vi "卫星模拟器自动控制软件.vi"() -> ()   [LabVIEW 2012]
uses:
  <vilib>/Utility/error.llb/DialogType.ctl
  <vilib>/DAQmx/create/channels.llb/DAQmx Create Channel (DO-Digital Output).vi
  <vilib>/vision/NI_Vision_Development_Module.lvlib
panel:
  in  "缩放比例 (像素/cm)":dbl=4.099468
  in  "远程数据记录器传输状态":bool
  in  "是否下传定位点信息":bool
  in  "远程端口":u16=61557
  in  "本地端口":u16=61556
  in  "远程终端地址":string="localhost"
  in  "broadcast":bool
  in  "是否姿态保持":bool
  out "alpha":dbl
  out "定位点信息":T1(array[cluster]) {"Aspect Ratio" format="%.2f"; "Orientation" format="%.2f"; "Area" format="%.2f"; "Object Center"."Y" format="%.2f"; "Object Center"."X" format="%.2f"}
  in  "Y中心校正":dbl
  in  "X中心校正":dbl
  out "相对偏角(deg)":dbl
  in  "目标Y":dbl
  in  "目标X":dbl
  out "X速率(cm/s)":dbl
  out "Y速率(cm/s)":dbl
  in  "OK Button":bool
  out "角速度(deg/s)":dbl
  in  "气浮状态":bool
  in  "控制频率(Hz)":u32=20
  in  "目标偏角":dbl
  in  "STOP":bool caption="stop (F)"
  out "导航相机输出":T2(plugin-control)
  out "alpha (deg)":dbl
  out "X偏移量 (cm)":dbl
  out "Y偏移量 (cm)":dbl
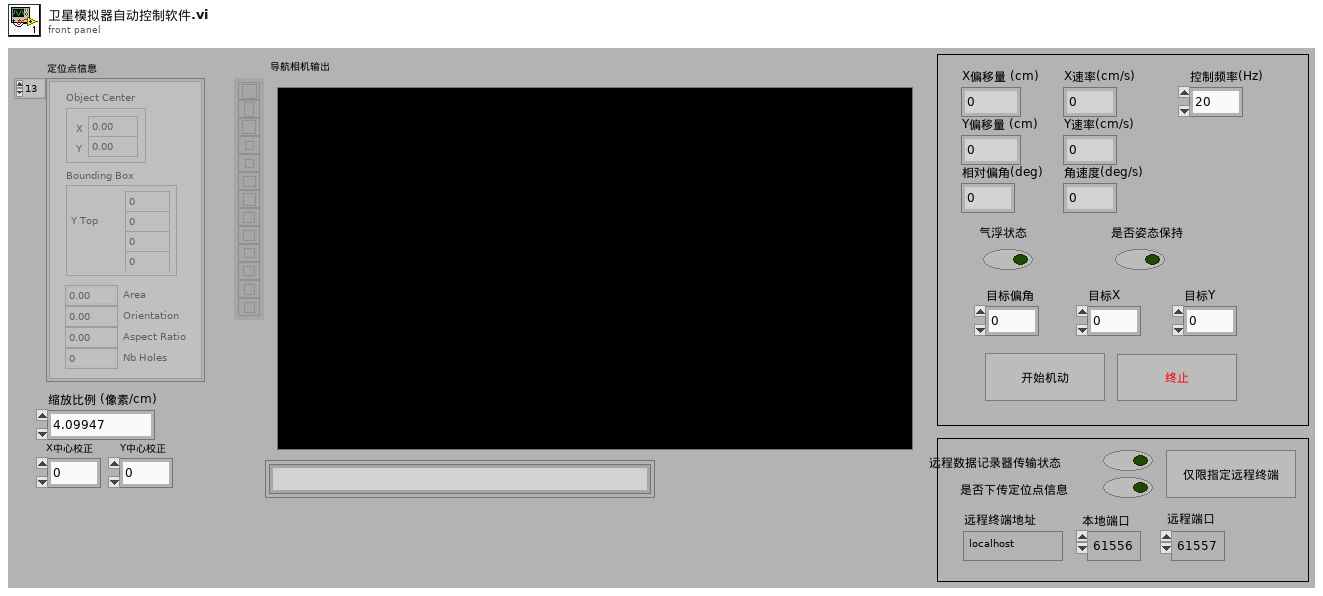
[diagram p1: front panel]
types:
  T1 = cluster{"Object Center":cluster{"X":sgl, "Y":sgl}, "Bounding Box":cluster{"X Left":i32, "Y Top":i32, "X Right":i32, "Y Bottom":i32}, "Area":sgl, "Orientation":sgl, "Aspect Ratio":sgl, "Nb Holes":i32}[]
  T2 = typedef "IMAQ Image.ctl" = refnum<image>
  T3 = typedef "DialogType.ctl" = u16
  T4 = cluster{"X偏移量 (cm)":dbl, "Y偏移量 (cm)":dbl, "相对偏角(deg)":dbl}
  T5 = cluster{"Objects":u16, "Threshold":i32, "Reject Border":bool, "Fill Holes":bool, "Min Object Size":bool, "Min Size":i32, "Max Object Size":bool, "Max Size":i32, "Show Search Area":bool, "Show Center":bool, "Show Bounding Box":bool}
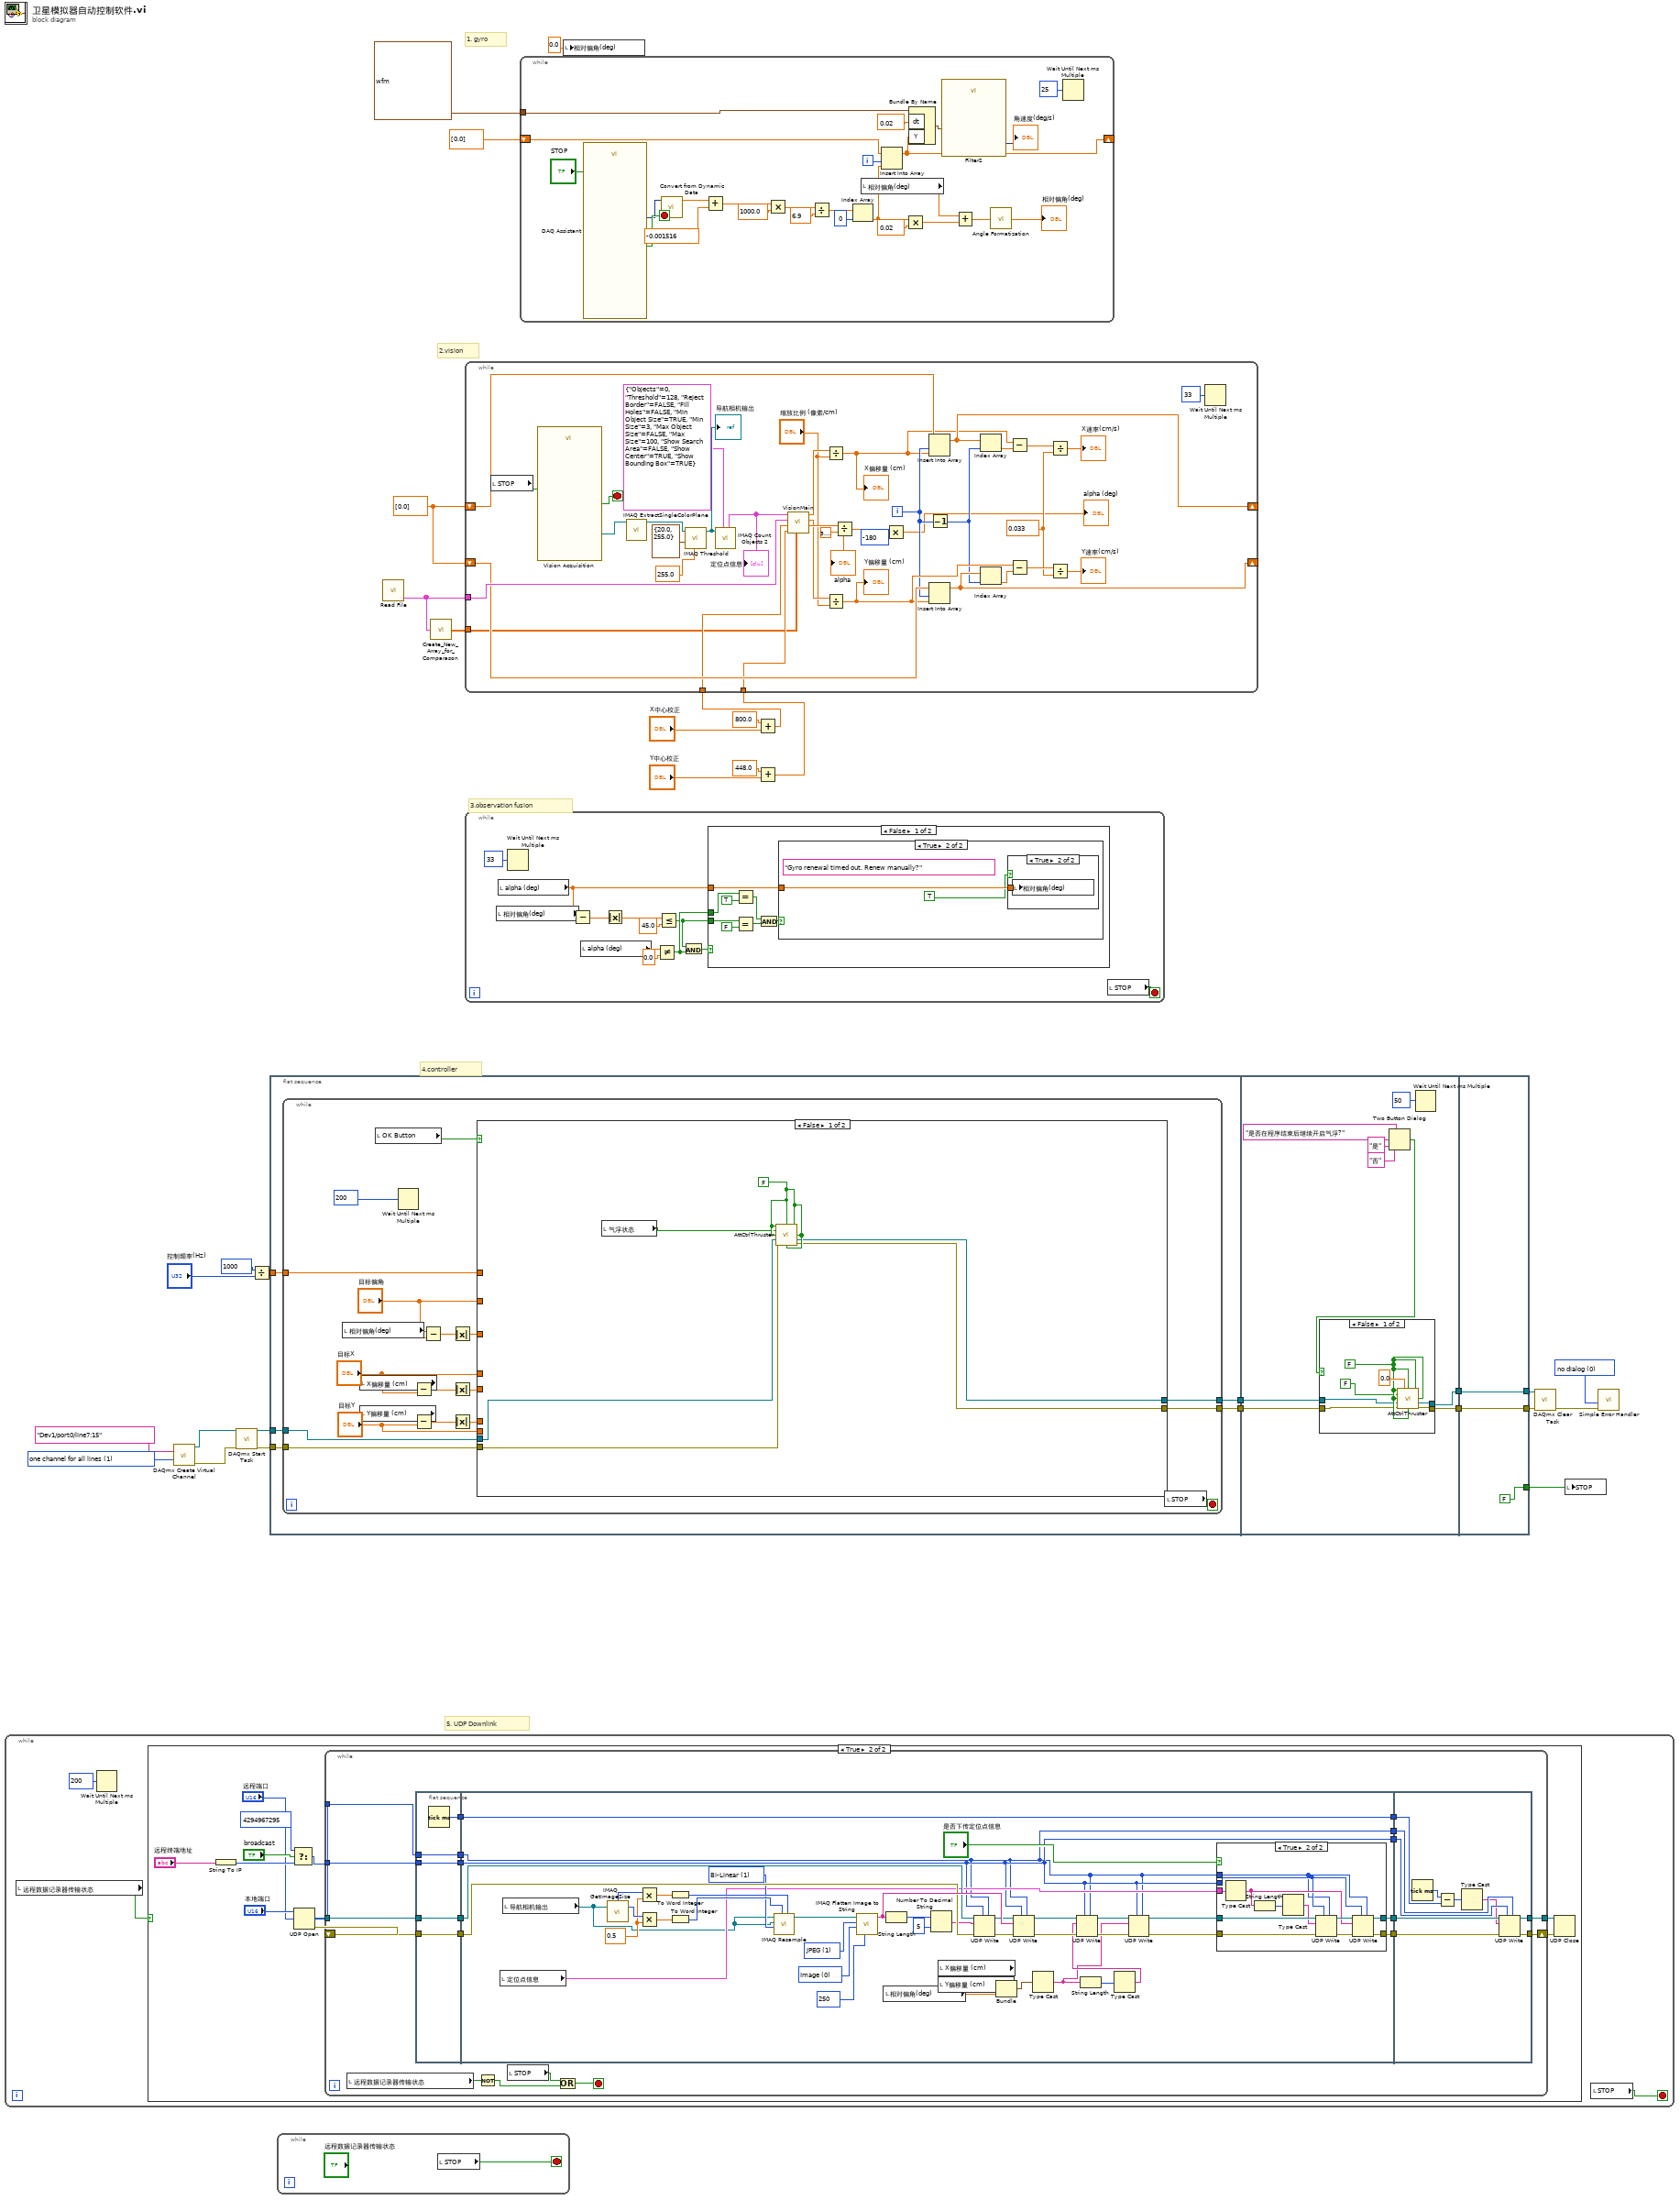
[diagram p0: block diagram]
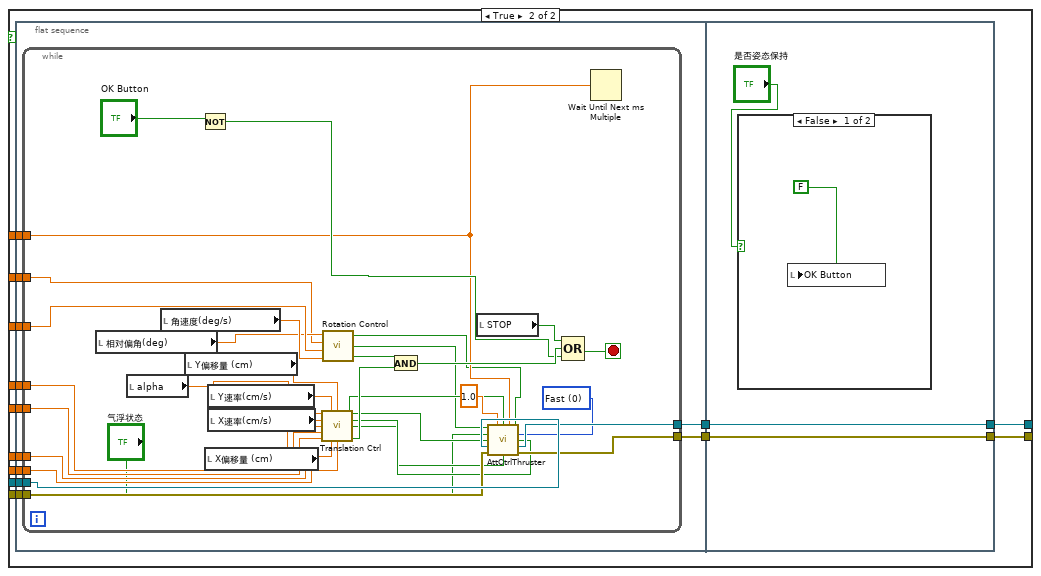
[diagram p4: hidden frame]
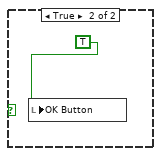
[diagram p5: hidden frame]
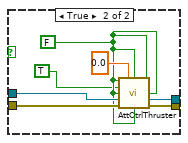
[diagram p6: hidden frame]
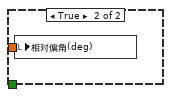
[diagram p9: hidden frame]
diagram:
  w25 = T3 0 items=["no dialog", "OK message", "continue or stop message", "OK message + warnings", "continue/stop + warnings"] ("type of dialog (OK msg:1)")
  w28 = 1 items=["one channel for each line", "one channel for all lines"] ("line grouping")
  w12 = dbl[] [0.0]
  # "5. UDP Downlink"
  # "4.controller"
  # "3.observation fusion"
  # "2.vision"
  # "1. gyro"
  n1 = while {
    stop <- w32 stop-if-true
    n2 = local read "远程数据记录器传输状态"() -> (w33:bool)
    n3 = Wait Until Next ms Multiple(millisecond multiple=u32 200) -> ()  [unwired: 1 out]
    n4 = case shown="True" w33 {
      frame False {
      }
      frame True {
        n5 = String To IP(1:"远程终端地址") -> (0:w41:u32)
        n6 = Select(t=u32 4294967295, s="broadcast", f=w41) -> (s? t:f=w38:u32)
        n7 = UDP Open(11:"本地端口") -> (port=w37:refnum<k16>, 0:w36:errorcluster)  [unwired: 1 in, 4 out]
        n8 = while {
          tunnel: "远程端口" -> [w64]
          tunnel: w38 -> [w63]
          tunnel: w37 -> [w62]
          tunnel: [w60] -> w35
          shift-right: [w59] -> w34
          shift-left: w36 -> [w61]
          stop <- w48 stop-if-true
          n9 = local read "远程数据记录器传输状态"() -> (w46:bool)
          n10 = flat-sequence {
            tunnel: w62 -> [w66]
            tunnel: w64 -> [w67]
            tunnel: w63 -> [w68]
            tunnel: w61 -> [w69]
            tunnel: [w69] -> w58
            tunnel: [w68] -> w57
            tunnel: [w67] -> w56
            tunnel: [w66] -> w55
            tunnel: [w65] -> w54
            tunnel: [w89] -> w53
            tunnel: [w88] -> w52
            tunnel: w58 -> [w107]
            tunnel: w57 -> [w71]
            tunnel: w56 -> [w70]
            tunnel: w55 -> [w91]
            tunnel: [w90] -> w51
            tunnel: w54 -> [w90]
            tunnel: [w70] -> w50
            tunnel: [w71] -> w49
            tunnel: [w131] -> w60
            tunnel: [w125] -> w59
            tunnel: w53 -> [w126]
            tunnel: w52 -> [w132]
            tunnel: w51 -> [w133]
            tunnel: w50 -> [w130]
            tunnel: w49 -> [w129]
            frame #0 {
              n11 = Tick Count (ms)() -> (millisecond timer value=w65:u32)
            }
            frame #1 {
              w95 = u32 1 items=["Zero Order", "Bi-Linear", "Quadratic", "Cubic Spline"] ("Interpolation Type")
              w96 = 0.5
              w104 = 0 items=["Image", "Image and Vision Info", "Reference to Image"] ("Type of Flatten (Image and Vision Info)")
              w109 = 1 items=["None", "JPEG", "PACKED BINARY"] ("Compression (None)")
              n12 = local read "定位点信息"() -> (w86:T1)
              n13 = local read "导航相机输出"() -> (w85:T2)
              n14 = call "IMAQ GetImageSize"("Image"=w85) -> ("Y Resolution"=w97:i32, "X Resolution"=w98:i32)  [unwired: 3 in, 1 out]
              n15 = Multiply(x=w98, y=w96) -> (x*y=w100:dbl)
              n16 = Multiply(x=w97, y=w96) -> (x*y=w102:dbl)
              n17 = To Word Integer(number=w100) -> (16bit integer=w99:i16)
              n18 = To Word Integer(number=w102) -> (16bit integer=w101:i16)
              n19 = call "IMAQ Resample"("X Resolution"=w99, "Y Resolution"=w101, "Interpolation Type"=w95, "Image Dst"=w85, "Image Src"=w85) -> ("Image Dst Out"=w103:T2)  [unwired: 5 in, 1 out]
              n20 = call "IMAQ Flatten Image to String"("Quality (750)"=250, "Type of Flatten (Image and Vision Info)"=w104, "Compression (None)"=w109, "Image"=w103) -> ("Data String"=w108:string)  [unwired: 6 in, 1 out]
              n21 = local read "相对偏角(deg)"() -> (w82:dbl)
              n22 = String Length(string=w108) -> (length=w94:i32)
              n23 = Number To Decimal String(number=w94, width (-)=i16 5) -> (decimal integer string=w93:string)
              n24 = local read "X偏移量 (cm)"() -> (w84:dbl)
              n25 = local read "Y偏移量 (cm)"() -> (w83:dbl)
              n26 = UDP Write(address=w71, port or service name=w70, connection ID=w91, data in=w93, 8:w107) -> (error out=w106:errorcluster, 3:w105:refnum<k16>)  [unwired: 1 out]
              n27 = Bundle("X偏移量 (cm)"=w84, "Y偏移量 (cm)"=w83, "相对偏角(deg)"=w82) -> (w81:T4)  [unwired: 1 in]
              n28 = UDP Write(address=w71, port or service name=w70, connection ID=w105, data in=w108, 8:w106) -> (error out=w79:errorcluster, 3:w80:refnum<k16>)  [unwired: 1 out]
              n29 = Type Cast(x=w81) -> (*(type *) &x=w72:string)  [unwired: 1 in]
              n30 = String Length(string=w72) -> (length=w74:i32)
              n31 = Type Cast(x=w74) -> (*(type *) &x=w73:string)  [unwired: 1 in]
              n32 = UDP Write(address=w71, port or service name=w70, connection ID=w80, data in=w73, 8:w79) -> (error out=w78:errorcluster, 3:w76:refnum<k16>)  [unwired: 1 out]
              n33 = UDP Write(address=w71, port or service name=w70, connection ID=w76, data in=w72, 8:w78) -> (error out=w77:errorcluster, 3:w75:refnum<k16>)  [unwired: 1 out]
              n34 = case shown="True" "是否下传定位点信息" {
                tunnel: w86 -> [_ w124]
                tunnel: w77 -> [w112 w122]
                tunnel: [w112 w120] -> w89
                tunnel: w75 -> [w111 w119]
                tunnel: [w111 w117] -> w88
                tunnel: w71 -> [_ w114]
                tunnel: w70 -> [_ w113]
                frame False {
                }
                frame True {
                  n35 = Type Cast(x=w124) -> (*(type *) &x=w115:string)  [unwired: 1 in]
                  n36 = String Length(string=w115) -> (length=w123:i32)
                  n37 = Type Cast(x=w123) -> (*(type *) &x=w116:string)  [unwired: 1 in]
                  n38 = UDP Write(address=w114, port or service name=w113, connection ID=w119, data in=w116, 8:w122) -> (error out=w121:errorcluster, 3:w118:refnum<k16>)  [unwired: 1 out]
                  n39 = UDP Write(address=w114, port or service name=w113, connection ID=w118, data in=w115, 8:w121) -> (error out=w120:errorcluster, 3:w117:refnum<k16>)  [unwired: 1 out]
                }
              }
            }
            frame #2 {
              n40 = Tick Count (ms)() -> (millisecond timer value=w134:u32)
              n41 = Subtract(x=w134, y=w133) -> (x-y=w128:u32)
              n42 = Type Cast(x=w128) -> (*(type *) &x=w127:string)  [unwired: 1 in]
              n43 = UDP Write(address=w129, port or service name=w130, connection ID=w132, data in=w127, 8:w126) -> (error out=w125:errorcluster, 3:w131:refnum<k16>)  [unwired: 1 out]
            }
          }
          n44 = Not(x=w46) -> (.not. x?=w45:bool)
          n45 = local read "STOP"() -> (w47:bool)
          n46 = Or(x=w47, y=w45) -> (x .or. y?=w48:bool)
        }
        n47 = UDP Close(connection ID=w35, 8:w34) -> ()  [unwired: 2 out]
      }
    }
    n48 = local read "STOP"() -> (w32:bool)
  }
  n49 = call-poly <vilib>:"DAQmx Create Virtual Channel.vi"("lines"=tag "Dev1/port0/line7:15" ("Lines"), "line grouping"=w28) -> ("task out"=w26:refnum<k21>, "error out"=w27:errorcluster)  [unwired: 12 in]
  n50 = call <vilib>:"DAQmx Start Task.vi"("task/channels in"=w26, "error in"=w27) -> ("task out"=w21:refnum<k21>, "error out"=w20:errorcluster)  [unwired: 12 in]
  n51 = Divide(x=u32 1000 ("milliseconds to wait"), y="控制频率(Hz)") -> (x/y=w17:dbl)
  n52 = flat-sequence {
    tunnel: w21 -> [w139]
    tunnel: w20 -> [w138]
    tunnel: w17 -> [w135]
    tunnel: [w137] -> w16
    tunnel: [w136] -> w15
    tunnel: w16 -> [w237]
    tunnel: w15 -> [w235]
    tunnel: [w236] -> w5
    tunnel: [w234] -> w4
    tunnel: [w253] -> w18
    tunnel: [w254] -> w19
    tunnel: w5 -> [w254]
    tunnel: w4 -> [w253]
    tunnel: [FALSE] -> w3
    frame #0 {
      n53 = while {
        tunnel: w139 -> [w159]
        tunnel: w138 -> [w158]
        tunnel: [w157] -> w137
        tunnel: [w156] -> w136
        tunnel: w135 -> [w141]
        stop <- w155 stop-if-true
        n54 = local read "相对偏角(deg)"() -> (w154:dbl)
        n55 = local read "X偏移量 (cm)"() -> (w150:dbl)
        n56 = local read "Y偏移量 (cm)"() -> (w146:dbl)
        n57 = local read "OK Button"() -> (w142:bool)
        n58 = Wait Until Next ms Multiple(millisecond multiple=200) -> ()  [unwired: 1 out]
        n59 = Subtract(x=w150, y="目标X") -> (x-y=w148:dbl)
        n60 = Subtract(x=w146, y="目标Y") -> (x-y=w144:dbl)
        n61 = Subtract(x=w154, y="目标偏角") -> (x-y=w152:dbl)
        n62 = Absolute Value(x=w152) -> (abs(x)=w151:dbl)
        n63 = Absolute Value(x=w148) -> (abs(x)=w147:dbl)
        n64 = Absolute Value(x=w144) -> (abs(x)=w143:dbl)
        n65 = case shown="False" w142 {
          tunnel: w159 -> [w163 w178]
          tunnel: w158 -> [w162 w177]
          tunnel: [w160 w176] -> w157
          tunnel: [w161 w175] -> w156
          tunnel: w141 -> [_ w174]
          tunnel: "目标偏角" -> [_ w173]
          tunnel: w151 -> [_ w172]
          tunnel: "目标X" -> [_ w171]
          tunnel: w147 -> [_ w170]
          tunnel: "目标Y" -> [_ w169]
          tunnel: w143 -> [_ w168]
          frame False {
            w165 = FALSE
            n66 = local read "气浮状态"() -> (w164:bool)
            n67 = call "AttCtrlThruster.vi"("ctclk"=w165, "Up"=w165, "clkwis"=w165, "Float"=w164, "Left"=w165, "Right"=w165, "task in"=w163, "error in"=w162, "Down"=w165) -> ("task out"=w161:refnum<k21>, "error out"=w160:errorcluster)  [unwired: 5 in]
          }
          frame True {
            n68 = flat-sequence {
              tunnel: w178 -> [w189]
              tunnel: w177 -> [w188]
              tunnel: w174 -> [w185]
              tunnel: w173 -> [w184]
              tunnel: w172 -> [w183]
              tunnel: w171 -> [w182]
              tunnel: w170 -> [w181]
              tunnel: w169 -> [w180]
              tunnel: w168 -> [w179]
              tunnel: [w187] -> w167
              tunnel: [w186] -> w166
              tunnel: [w225] -> w175
              tunnel: [w226] -> w176
              tunnel: w167 -> [w226]
              tunnel: w166 -> [w225]
              frame #0 {
                n69 = while {
                  tunnel: w189 -> [w223]
                  tunnel: w188 -> [w222]
                  tunnel: [w220] -> w187
                  tunnel: [w221] -> w186
                  tunnel: w185 -> [w193]
                  tunnel: w184 -> [w201]
                  tunnel: w183 -> [w216]
                  tunnel: w182 -> [w200]
                  tunnel: w181 -> [w211]
                  tunnel: w180 -> [w199]
                  tunnel: w179 -> [w198]
                  stop <- w217 stop-if-true
                  w207 = u16 0 items=["Fast", "Slow"] ("Angular Acceleration")
                  n70 = local read "相对偏角(deg)"() -> (w214:dbl)
                  n71 = local read "alpha"() -> (w195:dbl)
                  n72 = local read "角速度(deg/s)"() -> (w215:dbl)
                  n73 = local read "Y偏移量 (cm)"() -> (w209:dbl)
                  n74 = Not(x="OK Button") -> (.not. x?=w196:bool)
                  n75 = local read "X偏移量 (cm)"() -> (w212:dbl)
                  n76 = local read "Y速率(cm/s)"() -> (w210:dbl)
                  n77 = local read "X速率(cm/s)"() -> (w213:dbl)
                  n78 = call "Translation Ctrl.vi"("Alpha"=w195, "Filtered Speed Y"=w210, "Y In"=w209, "Filtered Speed X"=w213, "X In"=w212, "X Desired"=w200, "Original Difference X"=w211, "Original Difference Y"=w198, "Y Desired"=w199) -> ("Left"=w205:bool, "Right"=w204:bool, "Down"=w203:bool, "Up"=w202:bool, "Maneuver Complete?"=w206:bool)  [unwired: 2 in]
                  n79 = call "Rotation Control.vi"("Filtered Ohmega"=w215, "Original Difference"=w216, "Alpha Desired"=w201, "Alpha In"=w214) -> ("Maneuver Complete?"=w194:bool, "Counter-ClkWise Rot Ctrl"=w190:bool, "Clockwise Rot Ctrl"=w191:bool)
                  n80 = And(x=w194, y=w206) -> (x .and. y?=w208:bool)
                  n81 = local read "STOP"() -> (w218:bool)
                  n82 = call "AttCtrlThruster.vi"("ctclk"=w190, "Duty Cycle"=1.0, "Up"=w202, "Period"=w193, "clkwis"=w191, "Float"="气浮状态", "Angular Acceleration"=w207, "Left"=w205, "Right"=w204, "task in"=w223, "error in"=w222, "Down"=w203) -> ("task out"=w221:refnum<k21>, "error out"=w220:errorcluster)  [unwired: 2 in]
                  n83 = Compound Arithmetic op=OR(w218, w208, w196) -> (w217:bool)
                  n84 = Wait Until Next ms Multiple(millisecond multiple=w193) -> ()  [unwired: 1 out]
                }
              }
              frame #1 {
                n85 = case shown="False" "是否姿态保持" {
                  frame False {
                    n86 = local write "OK Button"(FALSE) -> ()
                  }
                  frame True {
                    n87 = local write "OK Button"(TRUE) -> ()
                  }
                }
              }
            }
          }
        }
        n88 = local read "STOP"() -> (w155:bool)
      }
    }
    frame #1 {
      n89 = Two Button Dialog(message="是否在程序结束后继续开启气浮?", 1:"否" ("F button name (\"Cancel\")"), 2:"是" ("T button name (\"OK\")")) -> (T button?=w231:bool)
      n90 = case shown="False" w231 {
        tunnel: w237 -> [w240 w251]
        tunnel: [w238 w250] -> w236
        tunnel: w235 -> [w241 w249]
        tunnel: [w239 w248] -> w234
        frame False {
          w243 = FALSE
          n91 = call "AttCtrlThruster.vi"("ctclk"=w243, "Duty Cycle"=0.0, "Up"=w243, "clkwis"=w243, "Float"=FALSE, "Left"=w243, "Right"=w243, "task in"=w241, "error in"=w240, "Down"=w243) -> ("task out"=w239:refnum<k21>, "error out"=w238:errorcluster)  [unwired: 4 in]
        }
        frame True {
          w246 = FALSE
          n92 = call "AttCtrlThruster.vi"("ctclk"=w246, "Duty Cycle"=0.0, "Up"=w246, "clkwis"=w246, "Float"=TRUE, "Left"=w246, "Right"=w246, "task in"=w249, "error in"=w251, "Down"=w246) -> ("task out"=w248:refnum<k21>, "error out"=w250:errorcluster)  [unwired: 4 in]
        }
      }
      n93 = Wait Until Next ms Multiple(millisecond multiple=u32 50) -> ()  [unwired: 1 out]
    }
    frame #2 {
    }
  }
  n94 = while {
    stop <- w255 stop-if-true
    n95 = local read "STOP"() -> (w255:bool)
  }
  n96 = call "Read File.vi"() -> ("Objects"=w2:T1)  [unwired: 1 in, 1 out]
  n97 = call "Create_New_Array_for_Comparason.vi"("Captured Plots"=w2) -> ("Generated Distance Array"=w1:dbl[][])
  n98 = while {
    stop <- w266 stop-if-true
    n99 = local read "相对偏角(deg)"() -> (w265:dbl)
    n100 = local read "alpha (deg)"() -> (w261:dbl)
    n101 = Wait Until Next ms Multiple(millisecond multiple=u32 33) -> ()  [unwired: 1 out]
    n102 = Subtract(x=w265, y=w261) -> (x-y=w264:dbl)
    n103 = local read "alpha (deg)"() -> (w259:dbl)
    n104 = Absolute Value(x=w264) -> (abs(x)=w263:dbl)
    n105 = Not Equal?(x=w259, y=0.0) -> (x != y?=w257:bool)
    n106 = Less Or Equal?(x=w263, y=45.0) -> (x <= y?=w256:bool)
    n107 = And(x=w256, y=w257) -> (x .and. y?=w260:bool)
    n108 = case shown="False" w260 {
      tunnel: w261 -> [w268 w279]
      tunnel: w257 -> [w270 _]
      tunnel: w256 -> [w269 _]
      frame False {
        n109 = Equal?(x=w270, y=TRUE) -> (x = y?=w274:bool)
        n110 = Equal?(x=w269, y=FALSE) -> (x = y?=w273:bool)
        n111 = And(x=w274, y=w273) -> (x .and. y?=w271:bool)
        n112 = case shown="True" w271 {
          tunnel: w268 -> [_ w277]
          frame False {
          }
          frame True {
            (unwired) "Gyro renewal timed out. Renew manually?" ("message")
            n113 = case shown="True" TRUE {
              tunnel: w277 -> [_ w278]
              frame False {
              }
              frame True {
                n114 = local write "相对偏角(deg)"(w278) -> ()
              }
            }
          }
        }
      }
      frame True {
        n115 = local write "相对偏角(deg)"(w279) -> ()
      }
    }
    n116 = local read "STOP"() -> (w266:bool)
  }
  n117 = while {
    shift-right: [w287] -> _
    shift-left: dbl[] [0.0] -> [w288]
    tunnel: waveform(dbl) {"t0"=timestamp(0 s since 1904-01-01), "dt"=1.0, "Y"=[]} ("waveform") -> [w285]
    i -> [w286]
    stop <- w303 stop-if-true
    n118 = call "DAQ Assistant"("stop (F)"="STOP") -> ("data"=w295:dynamicdata, "stopped"=w303:bool)  [unwired: 15 in, 2 out]
    n119 = call "Convert from Dynamic Data"("Dynamic Data Type"=w295) -> ("Array"=w293:dbl[])  [unwired: 3 in]
    n120 = Add(x=w293, y=-0.001516) -> (x+y=w291:dbl[])
    n121 = Multiply(x=w291, y=1000.0) -> (x*y=w302:dbl[])
    n122 = Divide(x=w302, y=6.9) -> (x/y=w296:dbl[])
    n123 = Index Array(array=w296, index=0) -> (element=w281:dbl)
    n124 = local read "相对偏角(deg)"() -> (w290:dbl)
    n125 = Insert Into Array(array=w288, index=w286, new element=w281) -> (w287:dbl[])
    n126 = Multiply(x=w281, y=0.02) -> (x*y=w297:dbl)
    n127 = Bundle By Name(cluster=w285, "dt"=0.02, "Y"=w287) -> (w284:waveform(dbl))
    n128 = call "Filter2"("Signal"=w284) -> ("Filtered Signal"=→"角速度(deg/s)":dynamicdata)  [unwired: 9 in, 1 out]
    n129 = Add(x=w290, y=w297) -> (x+y=w283:dbl)
    n130 = call "Angle Formatization.vi"("Alpha"=w283) -> ("Alpha Formatized"=→"相对偏角(deg)":dbl)
    n131 = Wait Until Next ms Multiple(millisecond multiple=u32 25 ("y")) -> ()  [unwired: 1 out]
  }
  n132 = local write "相对偏角(deg)"(0.0 ("y")) -> ()
  n133 = Add(x=800.0 ("c_x"), y="X中心校正") -> (x+y=w9:dbl)
  n134 = Add(x=448.0 ("c_y"), y="Y中心校正") -> (x+y=w6:dbl)
  n135 = while {
    tunnel: w2 -> [w330]
    shift-right: [w327] -> _
    shift-left: w12 -> [w328]
    shift-right: [w316] -> _
    shift-left: w12 -> [w319]
    tunnel: w6 -> [w309]
    tunnel: w9 -> [w308]
    tunnel: w1 -> [w305]
    i -> [w318]
    stop <- w341 stop-if-true
    w312 = 0.033 ("y")
    n136 = local read "STOP"() -> (w332:bool)
    n137 = call "Vision Acquisition"("Stop (F)"=w332) -> ("Image Out"=w336:T2, "Stopped"=w341:bool)  [unwired: 24 in, 1 out]
    n138 = call "IMAQ ExtractSingleColorPlane"("Image Src"=w336) -> ("Image Dst Out"=w340:T2)  [unwired: 9 in, 1 out]
    n139 = call "IMAQ Threshold"("Replace Value"=sgl 255.0 ("replace value"), "Range"=cluster{"lower value":sgl, "upper value":sgl} {"lower value"=20.0, "upper value"=255.0} ("threshold"), "Image Src"=w340) -> ("Image Dst Out"=w337:T2)  [unwired: 7 in, 1 out]
    "导航相机输出" <- w337
    n140 = call "IMAQ Count Objects 2"("Settings"=T5 {"Objects"=0, "Threshold"=128, "Reject Border"=FALSE, "Fill Holes"=FALSE, "Min Object Size"=TRUE, "Min Size"=3, "Max Object Size"=FALSE, "Max Size"=100, "Show Search Area"=FALSE, "Show Center"=TRUE, "Show Bounding Box"=TRUE}, "Image"=w337) -> ("Objects"=w331:T1)  [unwired: 5 in, 4 out]
    "定位点信息" <- w331
    n141 = call "VisionMain.vi"("Generated Distance Array"=w305, "Y Center"=w309, "X Center"=w308, "Original Plots"=w330, "Plots Captured"=w331) -> ("alpha"=w329:dbl, "dy"=w325:dbl, "dx"=w320:dbl)  [unwired: 4 in]
    "alpha" <- w329
    n142 = Divide(x=w320, y="缩放比例 (像素/cm)") -> (x/y=w315:dbl)
    "X偏移量 (cm)" <- w315
    n143 = Divide(x=w325, y="缩放比例 (像素/cm)") -> (x/y=w324:dbl)
    "Y偏移量 (cm)" <- w324
    n144 = Divide(x=w329, y=3.141592653589793) -> (x/y=w334:dbl)
    n145 = Multiply(x=w334, y=-180) -> (x*y=→"alpha (deg)":dbl)
    n146 = Insert Into Array(array=w319, index=w318, new element=w315) -> (w316:dbl[])
    n147 = Insert Into Array(array=w328, index=w318, new element=w324) -> (w327:dbl[])
    n148 = Decrement(x=w318) -> (x-1=w317:i32)
    n149 = Index Array(array=w316, index=w317) -> (element=w314:dbl)
    n150 = Index Array(array=w327, index=w317) -> (element=w326:dbl)
    n151 = Subtract(x=w315, y=w314) -> (x-y=w313:dbl)
    n152 = Subtract(x=w324, y=w326) -> (x-y=w323:dbl)
    n153 = Divide(x=w313, y=w312) -> (x/y=→"X速率(cm/s)":dbl)
    n154 = Divide(x=w323, y=w312) -> (x/y=→"Y速率(cm/s)":dbl)
    n155 = Wait Until Next ms Multiple(millisecond multiple=u32 33) -> ()  [unwired: 1 out]
  }
  n156 = call <vilib>:"DAQmx Clear Task.vi"("task in"=w18, "error in"=w19) -> ("error out"=w24:errorcluster)  [unwired: 13 in]
  n157 = local write "STOP"(w3) -> ()
  n158 = call <vilib>:"Simple Error Handler.vi"("type of dialog (OK msg:1)"=w25, "error in (no error)"=w24) -> ()  [unwired: 3 in, 5 out]
